vi "GenRasterScan.vi"() -> ()   [LabVIEW 2016]
uses:
  <vilib>/Math Plots/3D Math Plots/3D Scatter/3D Scatter XCtrl/3D Scatter.xctl
  <vilib>/Math Plots/3D Math Plots/3D Scatter/3D Scatter Datatype/Public/Plot Helper (Vector).vi
  <vilib>/Math Plots/3D Math Plots/3D Scatter/3D Scatter Datatype/3D Scatter Datatype.lvclass
panel:
  out "Task Space Trajectory":refnum<class "3D Plot Datatype.lvclass">[](xcontrol)
  in  "radius [mm]":dbl=3.0
  in  "dR [mm]":dbl=-0.5
  in  "Pmax [mm]":dbl=4.0
  in  "Vmax [mm/s]":dbl=4.0
  in  "Pad Length":i32=3000
  in  "Ts":dbl=0.001
  in  "nCycle":dbl=5.0
  in  "si":dbl[](array[numeric])=[0.0, 0.0, 0.0]
  in  "Stop":bool
  in  "Tab Control":T1(tab)
  out "Grooving Joint 1":dbl[](graph)
  out "Grooving Joint 2":dbl[](graph)
  out "Grooving Joint 3":dbl[](graph)
  in  "Generate Grooving":bool
  in  "Generate PC Mdl":bool
  in  "SCAN_NO":string="0004"
  out "Error IO":errorcluster
  in  "Generate Polishing Traj":bool
  in  "Matlab plot":bool=TRUE
  out "Joint 1":dbl[](graph)
  out "Joint 2":dbl[](graph)
  out "Joint 3":dbl[](graph)
  out "ILC Joint 3":dbl[](graph)
  out "ILC Joint 2":dbl[](graph)
  out "ILC Joint 1":dbl[](graph)
  in  "Generate ILC Trajectory":bool
  in  "Type":string(combo)="raster"
  in  "Generate Insertion":bool
  out "Insertion 1":dbl[](graph)
  out "Insertion 2":dbl[](graph)
  out "Insertion 3":dbl[](graph)
  out "ILC r":T2
  # "Parameters"
  # "x"
  # "y"
  # "z"
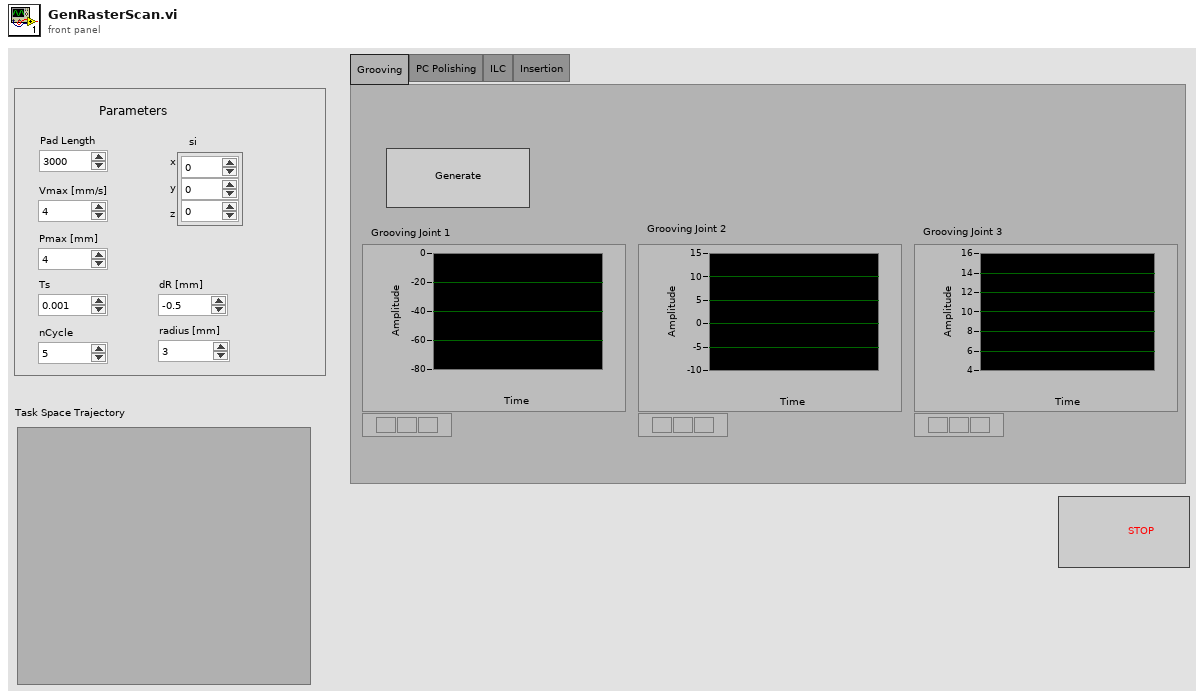
[diagram p1: front panel]
types:
  T1 = enum32{"Grooving", "PC Polishing", "ILC", "Insertion"}
  T2 = cluster{"Ref":cluster{"theta 1 Array":dbl[], "theta 2 Array":dbl[], "d3 Array":dbl[], "theta 4 Array":dbl[]}, "uFF":cluster{"theta 1 Array":dbl[], "theta 2 Array":dbl[], "d3 Array":dbl[], "theta 4 Array":dbl[]}, "yOut":cluster{"theta 1 Array":dbl[], "theta 2 Array":dbl[], "d3 Array":dbl[], "theta 4 Array":dbl[]}}
  T3 = cluster{"theta 1 Array":dbl[], "theta 2 Array":dbl[], "d3 Array":dbl[], "theta 4 Array":dbl[]}
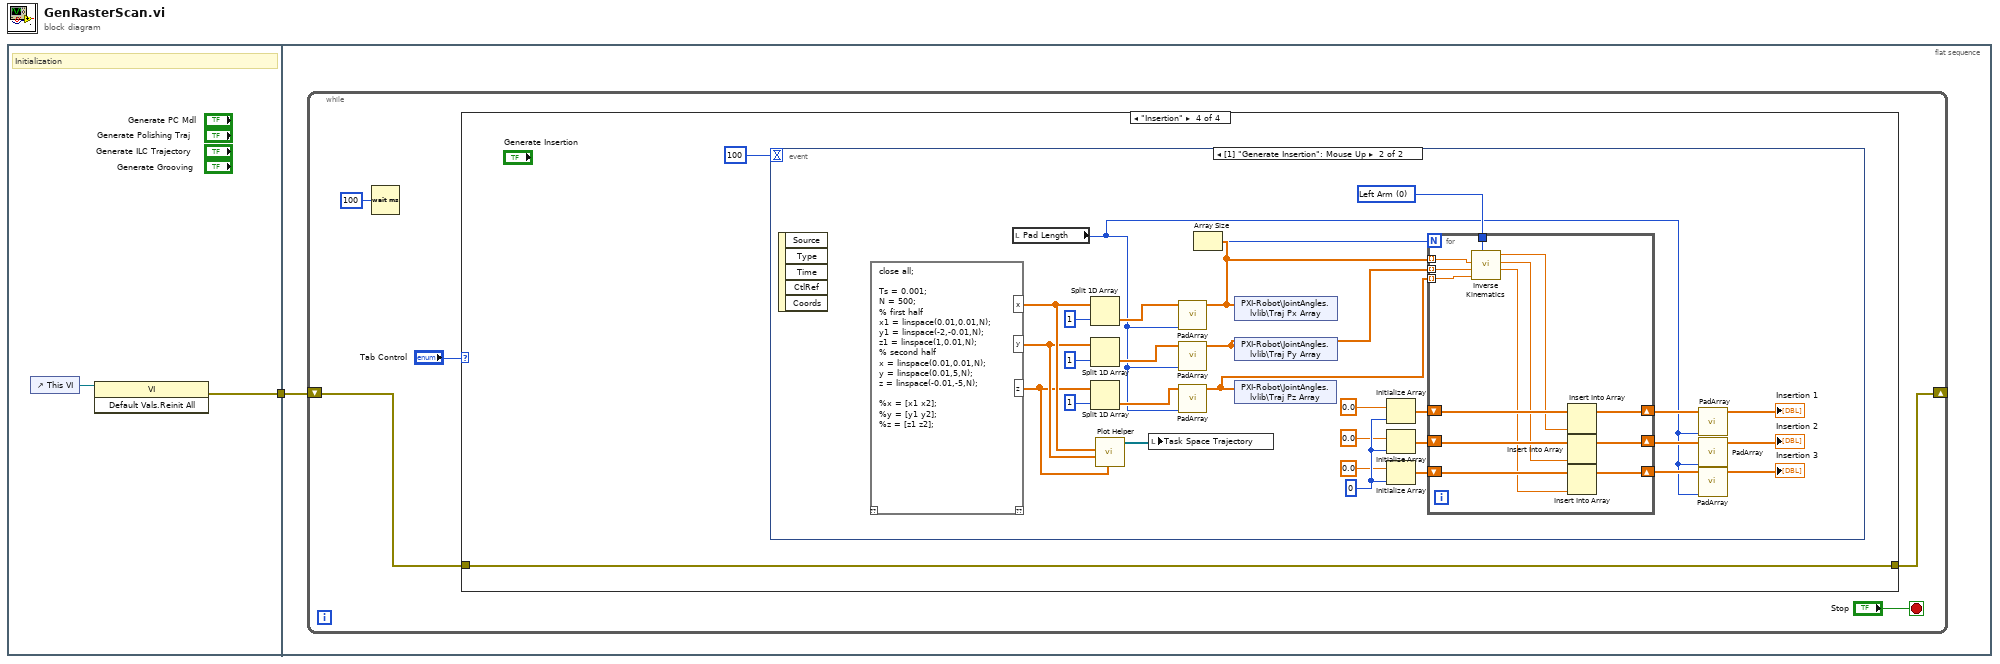
[diagram p0: block diagram]
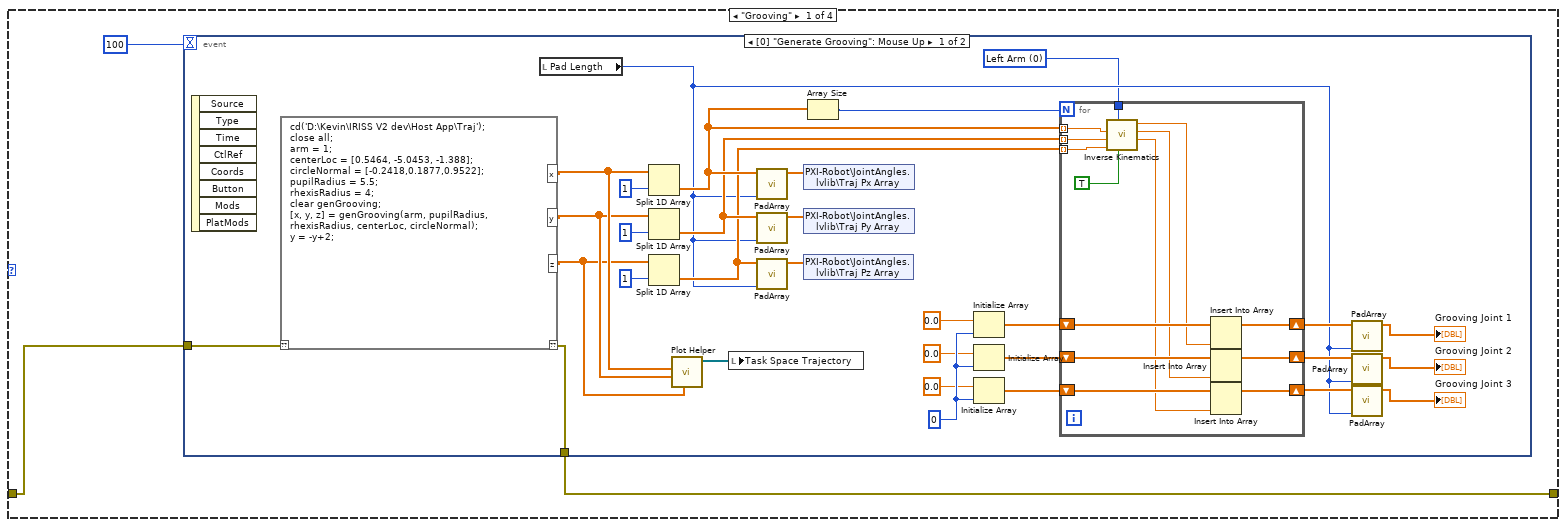
[diagram p2: hidden frame]
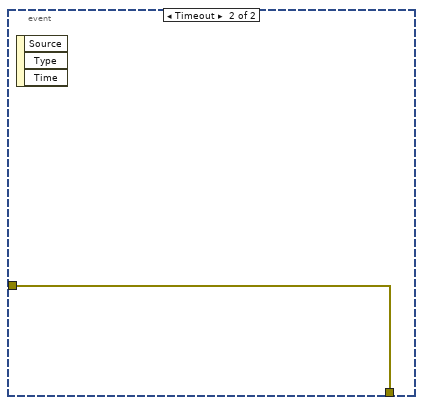
[diagram p3: hidden frame]
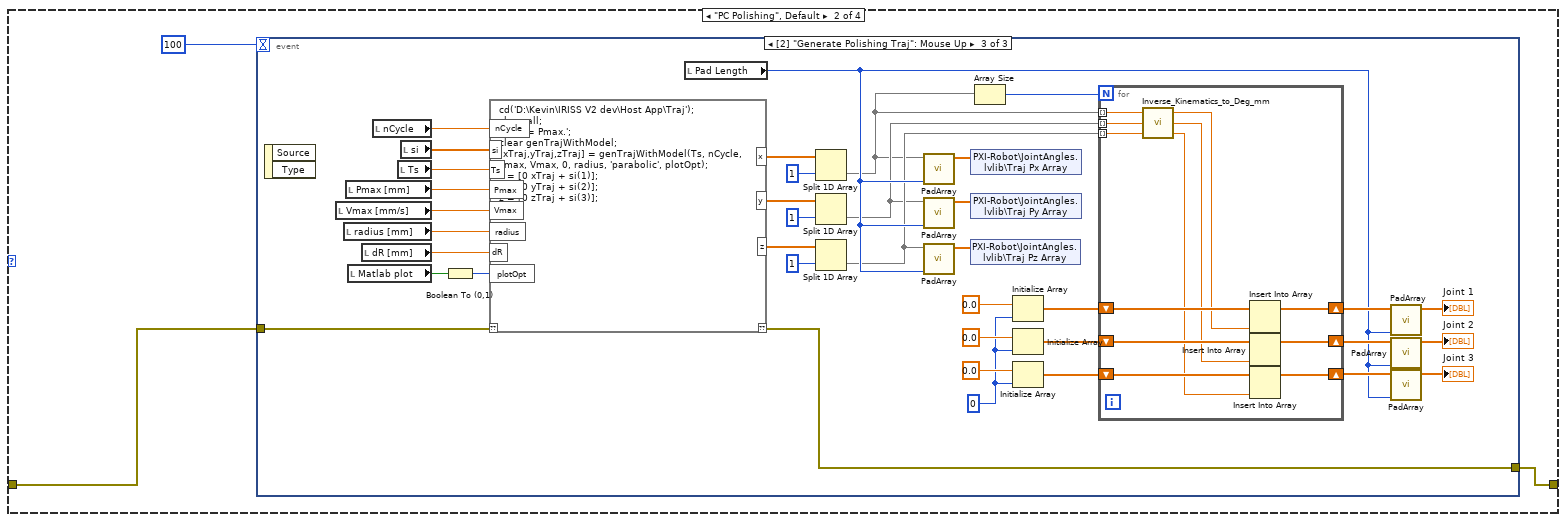
[diagram p4: hidden frame]
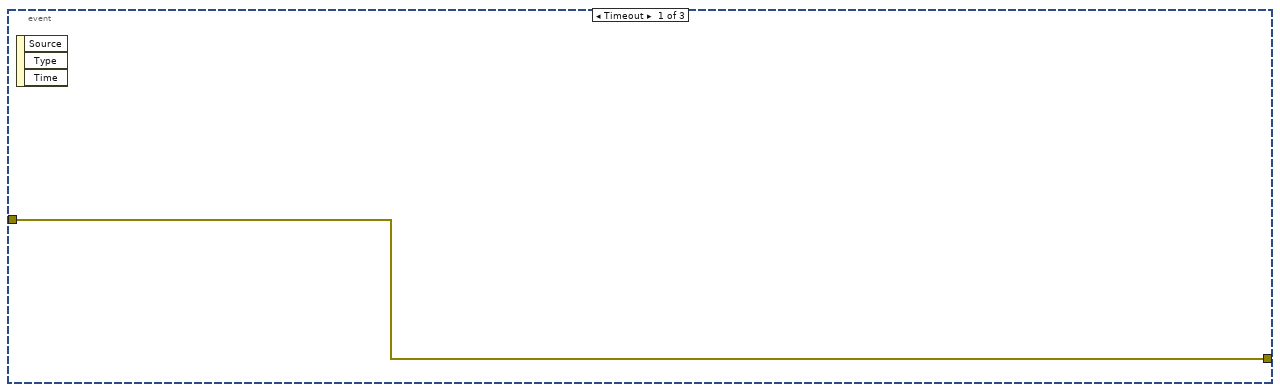
[diagram p5: hidden frame]
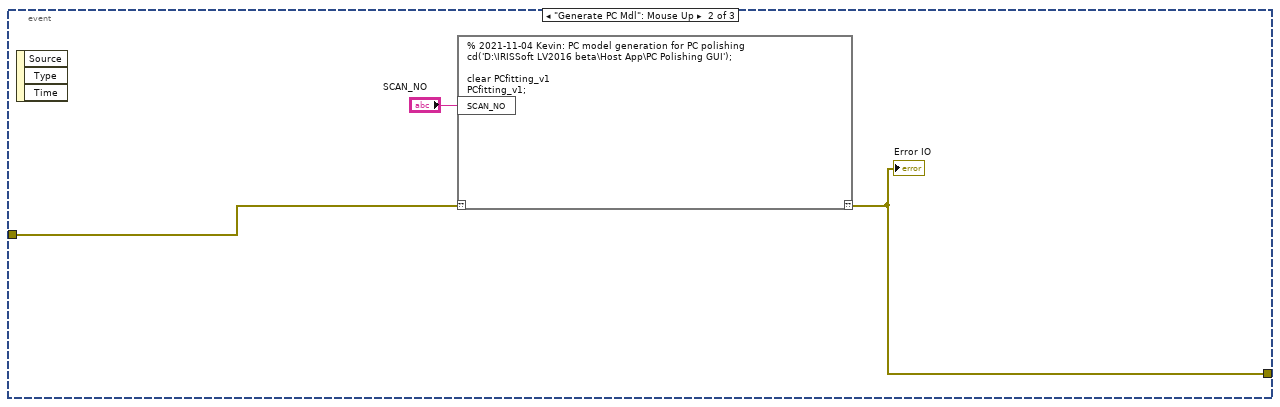
[diagram p6: hidden frame]
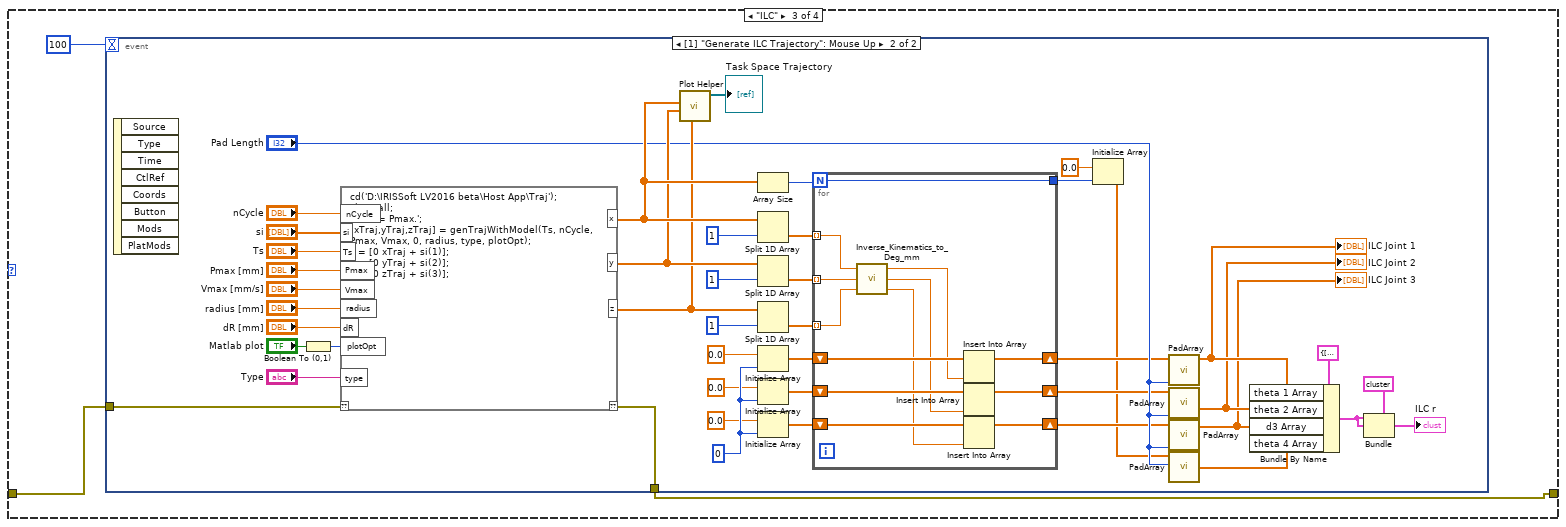
[diagram p7: hidden frame]
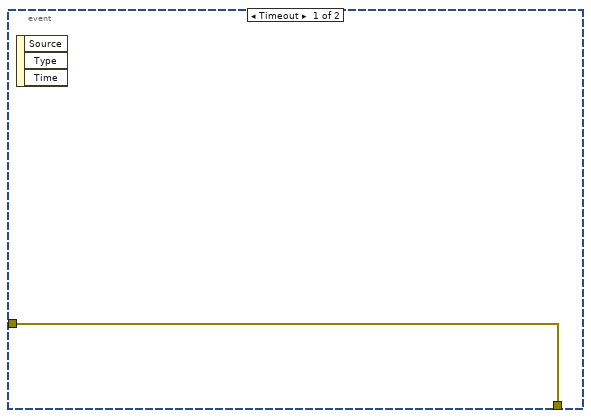
[diagram p8: hidden frame]
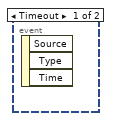
[diagram p9: hidden frame]
diagram:
  n1 = flat-sequence {
    tunnel: [w2] -> w1
    tunnel: w1 -> [w4]
    frame #0 {
      # "Initialization"
      n2 = control-ref of="This VI"() -> (w3:refnum<vi>)
      n3 = invoke class="VI" method="Default Vals.Reinit All"(reference=w3) -> (error out=w2:errorcluster)  [unwired: 2 in, 2 out]
    }
    frame #1 {
      n4 = while {
        shift-right: [w6] -> _
        shift-left: w4 -> [w7]
        stop <- "Stop" stop-if-true
        n5 = Wait (ms)(milliseconds to wait=u32 100) -> ()  [unwired: 1 out]
        n6 = case shown="\"Insertion\"" "Tab Control" {
          tunnel: w7 -> [w12 w60 w117 w179]
          tunnel: [w11 w59 w116 w179] -> w6
          frame "Grooving" {
            n7 = event shown="[0] \"Generate Grooving\": Mouse Up" {
              selector: _ -> [_ _]
              dyn-events: _ -> [_ _]
              timeout: 100 -> [_ _]
              tunnel: w12 -> [w18 w58]
              tunnel: [w17 w58] -> w11
              event "Generate Grooving": Mouse Up {
                w22 = 0 items=["Left Arm", "Right Arm"] ("armID")
                w31 = 0 ("dimension size")
                n8 = event-data() -> ()  [unwired: 1 in, 8 out]
                n9 = script code="cd('D:\\Kevin\\IRISS V2 dev\\Host App\\Traj');\nclose all;\narm = 1; \ncenterLoc = [0.5464, -5.0453, -1.388]; \ncircleNormal = [-0.2418,0.1877,0.9522]; \npupilRadius = 5.5; \nrhexisRadius = 4; \nclear genGrooving;\n[x, y, z] = genGrooving(arm, pupilRadius, rhexisRadius, centerLoc, circleNormal);\ny = -y+2;"("??"=w18) -> ("??"=w17:errorcluster, "x"=w15:dbl[], "y"=w14:dbl[], "z"=w13:dbl[])
                n10 = local read "Pad Length"() -> (w23:i32)
                n11 = Split 1D Array(array=w15, index=1) -> (second subarray=w26:dbl[])  [unwired: 1 out]
                n12 = Split 1D Array(array=w14, index=1) -> (second subarray=w25:dbl[])  [unwired: 1 out]
                n13 = Split 1D Array(array=w13, index=1) -> (second subarray=w24:dbl[])  [unwired: 1 out]
                n14 = call-poly <vilib>:"Plot Helper.vi"("z vector"=w13, "y vector"=w14, "x vector"=w15) -> ("3D Plot lvclass Array out"=w16:refnum<class "3D Plot Datatype.lvclass">[])  [unwired: 3 in, 5 out]
                n15 = local write "Task Space Trajectory"(w16) -> ()
                n16 = call "PadArray.vi"("Pad Length"=w23, "Input Array"=w26) -> ("Padded Array"=w41:dbl[])  [unwired: 9 in]
                n17 = call "PadArray.vi"("Pad Length"=w23, "Input Array"=w25) -> ("Padded Array"=w42:dbl[])  [unwired: 9 in]
                n18 = call "PadArray.vi"("Pad Length"=w23, "Input Array"=w24) -> ("Padded Array"=w43:dbl[])  [unwired: 9 in]
                n19 = shared-variable "PXI-Robot\\JointAngles.lvlib\\Traj Px Array"(w41) -> ()  [unwired: 1 in, 1 out]
                n20 = shared-variable "PXI-Robot\\JointAngles.lvlib\\Traj Py Array"(w42) -> ()  [unwired: 1 in, 1 out]
                n21 = shared-variable "PXI-Robot\\JointAngles.lvlib\\Traj Pz Array"(w43) -> ()  [unwired: 1 in, 1 out]
                n22 = Array Size(array=w26) -> (size(s)=w27:i32)
                n23 = Initialize Array(0.0 ("element"), w31) -> (w32:dbl[])
                n24 = Initialize Array(0.0 ("element"), w31) -> (w33:dbl[])
                n25 = Initialize Array(0.0 ("element"), w31) -> (w34:dbl[])
                n26 = for {
                  N: w27 -> [_]
                  tunnel: w26 -> [w50] mode=indexing
                  tunnel: w25 -> [w49] mode=indexing
                  tunnel: w24 -> [w48] mode=indexing
                  shift-right: [w56] -> w35
                  shift-left: w32 -> [w57]
                  shift-right: [w54] -> w36
                  shift-left: w33 -> [w55]
                  shift-right: [w52] -> w37
                  shift-left: w34 -> [w53]
                  tunnel: w22 -> [w51]
                  n27 = call "Inverse Kinematics.vi"("isToolTipInsideEye"=TRUE, "armID"=w51, "z"=w48, "y"=w49, "x"=w50) -> ("j3"=w45:dbl, "j2"=w46:dbl, "j1"=w47:dbl)  [unwired: 3 in, 1 out]
                  n28 = Insert Into Array(array=w57, new element=w47) -> (w56:dbl[])  [unwired: 1 in]
                  n29 = Insert Into Array(array=w55, new element=w46) -> (w54:dbl[])  [unwired: 1 in]
                  n30 = Insert Into Array(array=w53, new element=w45) -> (w52:dbl[])  [unwired: 1 in]
                }
                n31 = call "PadArray.vi"("Pad Length"=w23, "Input Array"=w35) -> ("Padded Array"=→"Grooving Joint 1":dbl[])  [unwired: 9 in]
                n32 = call "PadArray.vi"("Pad Length"=w23, "Input Array"=w36) -> ("Padded Array"=→"Grooving Joint 2":dbl[])  [unwired: 9 in]
                n33 = call "PadArray.vi"("Pad Length"=w23, "Input Array"=w37) -> ("Padded Array"=→"Grooving Joint 3":dbl[])  [unwired: 9 in]
              }
              event Timeout {
                n34 = event-data() -> ()  [unwired: 1 in, 3 out]
              }
            }
          }
          frame "PC Polishing", Default {
            n35 = event shown="[2] \"Generate Polishing Traj\": Mouse Up" {
              selector: _ -> [_ _ _]
              dyn-events: _ -> [_ _ _]
              timeout: 100 -> [_ _ _]
              tunnel: w60 -> [w62 w64 w102]
              tunnel: [w62 w63 w103] -> w59
              event Timeout {
                n36 = event-data() -> ()  [unwired: 1 in, 3 out]
              }
              event "Generate PC Mdl": Mouse Up {
                n37 = event-data() -> ()  [unwired: 1 in, 3 out]
                n38 = script code="% 2021-11-04 Kevin: PC model generation for PC polishing\ncd('D:\\IRISSoft LV2016 beta\\Host App\\PC Polishing GUI');\n\nclear PCfitting_v1\nPCfitting_v1;"("??"=w64, "SCAN_NO"="SCAN_NO") -> ("??"=w63:errorcluster)
                "Error IO" <- w63
              }
              event "Generate Polishing Traj": Mouse Up {
                w80 = 0 ("dimension size")
                n39 = event-data() -> ()  [unwired: 1 in, 2 out]
                n40 = local read "Vmax [mm/s]"() -> (w94:dbl)
                n41 = local read "radius [mm]"() -> (w95:dbl)
                n42 = local read "Pmax [mm]"() -> (w93:dbl)
                n43 = local read "Matlab plot"() -> (w98:bool)
                n44 = local read "dR [mm]"() -> (w96:dbl)
                n45 = local read "nCycle"() -> (w101:dbl)
                n46 = local read "Ts"() -> (w99:dbl)
                n47 = local read "si"() -> (w100:dbl[])
                n48 = Boolean To (0,1)(Boolean=w98) -> (0, 1=w97:i16)
                n49 = script code="cd('D:\\Kevin\\IRISS V2 dev\\Host App\\Traj');\nclose all;\nPmax = Pmax.';\nclear genTrajWithModel;\n[xTraj,yTraj,zTraj] = genTrajWithModel(Ts, nCycle, Pmax, Vmax, 0, radius, 'parabolic', plotOpt);\nx = [0 xTraj + si(1)];\ny = [0 yTraj + si(2)];\nz = [0 zTraj + si(3)];"("??"=w102, "nCycle"=w101, "Ts"=w99, "Vmax"=w94, "Pmax"=w93, "plotOpt"=w97, "si"=w100, "radius"=w95, "dR"=w96) -> ("??"=w103:errorcluster, "x"=w87:dbl[], "y"=w89:dbl[], "z"=w88:dbl[])
                n50 = local read "Pad Length"() -> (w72:i32)
                n51 = Split 1D Array(array=w87, index=1) -> (second subarray=w66:dbl[])  [unwired: 1 out]
                n52 = Split 1D Array(array=w89, index=1) -> (second subarray=w67:dbl[])  [unwired: 1 out]
                n53 = Split 1D Array(array=w88, index=1) -> (second subarray=w68:dbl[])  [unwired: 1 out]
                n54 = call "PadArray.vi"("Pad Length"=w72, "Input Array"=w66) -> ("Padded Array"=w86:dbl[])  [unwired: 9 in]
                n55 = call "PadArray.vi"("Pad Length"=w72, "Input Array"=w67) -> ("Padded Array"=w85:dbl[])  [unwired: 9 in]
                n56 = call "PadArray.vi"("Pad Length"=w72, "Input Array"=w68) -> ("Padded Array"=w84:dbl[])  [unwired: 9 in]
                n57 = shared-variable "PXI-Robot\\JointAngles.lvlib\\Traj Px Array"(w86) -> ()  [unwired: 1 in, 1 out]
                n58 = shared-variable "PXI-Robot\\JointAngles.lvlib\\Traj Py Array"(w85) -> ()  [unwired: 1 in, 1 out]
                n59 = shared-variable "PXI-Robot\\JointAngles.lvlib\\Traj Pz Array"(w84) -> ()  [unwired: 1 in, 1 out]
                n60 = Array Size(array=w66) -> (size(s)=w76:i32)
                n61 = Initialize Array(0.0 ("element"), w80) -> (w79:dbl[])
                n62 = Initialize Array(0.0 ("element"), w80) -> (w78:dbl[])
                n63 = Initialize Array(0.0 ("element"), w80) -> (w77:dbl[])
                n64 = for {
                  N: w76 -> [_]
                  tunnel: w66 -> [w115] mode=indexing
                  tunnel: w67 -> [w114] mode=indexing
                  tunnel: w68 -> [w113] mode=indexing
                  shift-right: [w110] -> w75
                  shift-left: w79 -> [w112]
                  shift-right: [w107] -> w74
                  shift-left: w78 -> [w109]
                  shift-right: [w104] -> w73
                  shift-left: w77 -> [w106]
                  n65 = call "Inverse_Kinematics_to_Deg_mm.vi"("pz"=w113, "py"=w114, "px"=w115) -> ("L3 [mm]"=w105:dbl, "L2 [deg]"=w108:dbl, "L1 [deg]"=w111:dbl)
                  n66 = Insert Into Array(array=w112, new element=w111) -> (w110:dbl[])  [unwired: 1 in]
                  n67 = Insert Into Array(array=w109, new element=w108) -> (w107:dbl[])  [unwired: 1 in]
                  n68 = Insert Into Array(array=w106, new element=w105) -> (w104:dbl[])  [unwired: 1 in]
                }
                n69 = call "PadArray.vi"("Pad Length"=w72, "Input Array"=w75) -> ("Padded Array"=→"Joint 1":dbl[])  [unwired: 9 in]
                n70 = call "PadArray.vi"("Pad Length"=w72, "Input Array"=w74) -> ("Padded Array"=→"Joint 2":dbl[])  [unwired: 9 in]
                n71 = call "PadArray.vi"("Pad Length"=w72, "Input Array"=w73) -> ("Padded Array"=→"Joint 3":dbl[])  [unwired: 9 in]
              }
            }
          }
          frame "ILC" {
            n72 = event shown="[1] \"Generate ILC Trajectory\": Mouse Up" {
              selector: _ -> [_ _]
              dyn-events: _ -> [_ _]
              timeout: 100 -> [_ _]
              tunnel: w117 -> [w119 w160]
              tunnel: [w119 w159] -> w116
              event Timeout {
                n73 = event-data() -> ()  [unwired: 1 in, 3 out]
              }
              event "Generate ILC Trajectory": Mouse Up {
                w129 = 0 ("dimension size")
                n74 = event-data() -> ()  [unwired: 1 in, 8 out]
                n75 = Boolean To (0,1)(Boolean="Matlab plot") -> (0, 1=w158:i16)
                n76 = script code="cd('D:\\IRISSoft LV2016 beta\\Host App\\Traj');\nclose all;\nPmax = Pmax.';\n[xTraj,yTraj,zTraj] = genTrajWithModel(Ts, nCycle, Pmax, Vmax, 0, radius, type, plotOpt);\nx = [0 xTraj + si(1)];\ny = [0 yTraj + si(2)];\nz = [0 zTraj + si(3)];"("??"=w160, "nCycle"="nCycle", "Ts"="Ts", "Vmax"="Vmax [mm/s]", "Pmax"="Pmax [mm]", "plotOpt"=w158, "si"="si", "radius"="radius [mm]", "dR"="dR [mm]", "type"="Type") -> ("??"=w159:errorcluster, "x"=w164:dbl[], "y"=w163:dbl[], "z"=w162:dbl[])
                n77 = call-poly <vilib>:"Plot Helper.vi"("z vector"=w162, "y vector"=w163, "x vector"=w164) -> ("3D Plot lvclass Array out"=→"Task Space Trajectory":refnum<class "3D Plot Datatype.lvclass">[])  [unwired: 3 in, 5 out]
                n78 = Array Size(array=w164) -> (size(s)=w140:i32)
                n79 = Split 1D Array(array=w164, index=1) -> (second subarray=w146:dbl[])  [unwired: 1 out]
                n80 = Split 1D Array(array=w163, index=1) -> (second subarray=w147:dbl[])  [unwired: 1 out]
                n81 = Split 1D Array(array=w162, index=1) -> (second subarray=w145:dbl[])  [unwired: 1 out]
                n82 = Initialize Array(0.0 ("element"), w129) -> (w126:dbl[])
                n83 = Initialize Array(0.0 ("element"), w129) -> (w127:dbl[])
                n84 = Initialize Array(0.0 ("element"), w129) -> (w128:dbl[])
                n85 = for {
                  N: w140 -> [w166]
                  tunnel: w146 -> [w177] mode=indexing
                  tunnel: w147 -> [w176] mode=indexing
                  tunnel: w145 -> [w175] mode=indexing
                  shift-right: [w172] -> w141
                  shift-left: w126 -> [w174]
                  shift-right: [w169] -> w142
                  shift-left: w127 -> [w171]
                  shift-right: [w167] -> w143
                  shift-left: w128 -> [w168]
                  tunnel: [w166] -> w138
                  n86 = call "Inverse_Kinematics_to_Deg_mm.vi"("pz"=w175, "py"=w176, "px"=w177) -> ("L3 [mm]"=w165:dbl, "L2 [deg]"=w170:dbl, "L1 [deg]"=w173:dbl)
                  n87 = Insert Into Array(array=w174, new element=w173) -> (w172:dbl[])  [unwired: 1 in]
                  n88 = Insert Into Array(array=w171, new element=w170) -> (w169:dbl[])  [unwired: 1 in]
                  n89 = Insert Into Array(array=w168, new element=w165) -> (w167:dbl[])  [unwired: 1 in]
                }
                n90 = Initialize Array(0.0 ("element"), w138) -> (w139:dbl[])
                n91 = call "PadArray.vi"("Pad Length"="Pad Length", "Input Array"=w141) -> ("Padded Array"=w122:dbl[])  [unwired: 9 in]
                "ILC Joint 1" <- w122
                n92 = call "PadArray.vi"("Pad Length"="Pad Length", "Input Array"=w142) -> ("Padded Array"=w121:dbl[])  [unwired: 9 in]
                "ILC Joint 2" <- w121
                n93 = call "PadArray.vi"("Pad Length"="Pad Length", "Input Array"=w143) -> ("Padded Array"=w120:dbl[])  [unwired: 9 in]
                "ILC Joint 3" <- w120
                n94 = call "PadArray.vi"("Pad Length"="Pad Length", "Input Array"=w139) -> ("Padded Array"=w144:dbl[])  [unwired: 9 in]
                n95 = Bundle By Name(cluster=T3 {"theta 1 Array"=[], "theta 2 Array"=[], "d3 Array"=[], "theta 4 Array"=[]} ("uFF"), "theta 1 Array"=w122, "theta 2 Array"=w121, "d3 Array"=w120, "theta 4 Array"=w144) -> (w134:T3)
                n96 = Bundle(cluster=T2 {"Ref"={"theta 1 Array"=array[6000 elements], "theta 2 Array"=array[6000 elements], "d3 Array"=array[6000 elements], "theta 4 Array"=array[6000 elements]}, "uFF"={"theta 1 Array"=array[6000 elements], "theta 2 Array"=array[6000 elements], "d3 Array"=array[6000 elements], "theta 4 Array"=array[6000 elements]}, "yOut"={"theta 1 Array"=[], "theta 2 Array"=[], "d3 Array"=[], "theta 4 Array"=[]}} ("Cluster"), "Ref"=w134, "uFF"=w134) -> (→"ILC r":T2)  [unwired: 1 in]
              }
            }
          }
          frame "Insertion" {
            n97 = event shown="[1] \"Generate Insertion\": Mouse Up" {
              selector: _ -> [_ _]
              dyn-events: _ -> [_ _]
              timeout: 100 -> [_ _]
              event Timeout {
                n98 = event-data() -> ()  [unwired: 1 in, 3 out]
              }
              event "Generate Insertion": Mouse Up {
                w182 = 0 items=["Left Arm", "Right Arm"] ("armID")
                w193 = 0 ("dimension size")
                n99 = event-data() -> ()  [unwired: 1 in, 5 out]
                n100 = script code="close all;\n\nTs = 0.001;\nN = 500;\n% first half\nx1 = linspace(0.01,0.01,N);\ny1 = linspace(-2,-0.01,N);\nz1 = linspace(1,0.01,N);\n% second half\nx = linspace(0.01,0.01,N);\ny = linspace(0.01,5,N);\nz = linspace(-0.01,-5,N);\n\n%x = [x1 x2];\n%y = [y1 y2];\n%z = [z1 z2];"() -> ("x"=w203:dbl[], "y"=w202:dbl[], "z"=w201:dbl[])  [unwired: 1 in, 1 out]
                n101 = local read "Pad Length"() -> (w181:i32)
                n102 = Split 1D Array(array=w203, index=1) -> (second subarray=w186:dbl[])  [unwired: 1 out]
                n103 = Split 1D Array(array=w202, index=1) -> (second subarray=w205:dbl[])  [unwired: 1 out]
                n104 = Split 1D Array(array=w201, index=1) -> (second subarray=w204:dbl[])  [unwired: 1 out]
                n105 = call-poly <vilib>:"Plot Helper.vi"("z vector"=w201, "y vector"=w202, "x vector"=w203) -> ("3D Plot lvclass Array out"=w200:refnum<class "3D Plot Datatype.lvclass">[])  [unwired: 3 in, 5 out]
                n106 = local write "Task Space Trajectory"(w200) -> ()
                n107 = call "PadArray.vi"("Pad Length"=w181, "Input Array"=w186) -> ("Padded Array"=w184:dbl[])  [unwired: 9 in]
                n108 = call "PadArray.vi"("Pad Length"=w181, "Input Array"=w205) -> ("Padded Array"=w185:dbl[])  [unwired: 9 in]
                n109 = call "PadArray.vi"("Pad Length"=w181, "Input Array"=w204) -> ("Padded Array"=w183:dbl[])  [unwired: 9 in]
                n110 = Array Size(array=w184) -> (size(s)=w180:i32)
                n111 = shared-variable "PXI-Robot\\JointAngles.lvlib\\Traj Px Array"(w184) -> ()  [unwired: 1 in, 1 out]
                n112 = shared-variable "PXI-Robot\\JointAngles.lvlib\\Traj Py Array"(w185) -> ()  [unwired: 1 in, 1 out]
                n113 = shared-variable "PXI-Robot\\JointAngles.lvlib\\Traj Pz Array"(w183) -> ()  [unwired: 1 in, 1 out]
                n114 = Initialize Array(0.0 ("element"), w193) -> (w194:dbl[])
                n115 = Initialize Array(0.0 ("element"), w193) -> (w195:dbl[])
                n116 = Initialize Array(0.0 ("element"), w193) -> (w196:dbl[])
                n117 = for {
                  N: w180 -> [_]
                  tunnel: w184 -> [w214] mode=indexing
                  tunnel: w185 -> [w213] mode=indexing
                  tunnel: w183 -> [w212] mode=indexing
                  shift-right: [w220] -> w197
                  shift-left: w194 -> [w221]
                  shift-right: [w218] -> w198
                  shift-left: w195 -> [w219]
                  shift-right: [w216] -> w199
                  shift-left: w196 -> [w217]
                  tunnel: w182 -> [w215]
                  n118 = call "Inverse Kinematics.vi"("armID"=w215, "z"=w212, "y"=w213, "x"=w214) -> ("j3"=w209:dbl, "j2"=w210:dbl, "j1"=w211:dbl)  [unwired: 4 in, 1 out]
                  n119 = Insert Into Array(array=w221, new element=w211) -> (w220:dbl[])  [unwired: 1 in]
                  n120 = Insert Into Array(array=w219, new element=w210) -> (w218:dbl[])  [unwired: 1 in]
                  n121 = Insert Into Array(array=w217, new element=w209) -> (w216:dbl[])  [unwired: 1 in]
                }
                n122 = call "PadArray.vi"("Pad Length"=w181, "Input Array"=w197) -> ("Padded Array"=→"Insertion 1":dbl[])  [unwired: 9 in]
                n123 = call "PadArray.vi"("Pad Length"=w181, "Input Array"=w198) -> ("Padded Array"=→"Insertion 2":dbl[])  [unwired: 9 in]
                n124 = call "PadArray.vi"("Pad Length"=w181, "Input Array"=w199) -> ("Padded Array"=→"Insertion 3":dbl[])  [unwired: 9 in]
              }
            }
          }
        }
      }
    }
  }
